vi "DMM_Scan PMPS 16V-15C Configure and Measure.vi"(0 "Scan Resources Handles In":T1, 5 "Scan Configuration":T5[](array[typedef]) {"Resolution in Digits" items=["3 1/2"=3.5, "4 1/2"=4.5, "5 1/2"=5.5, "6 1/2"=6.5, "7 1/2"=7.5]}, 11 "error in":errorcluster) -> (4 "Scan Resources Handles Out":T2, 6 "Formatted Measurements":T4[](array[typedef]) {"Switch Time" format="%#_3p"}, 8 "Raw Measurements":T3[](array[typedef]) {"Value" format="%#_8g"}, 10 "Execution Settings":T7[](array[typedef]) {"Function" items=["DC Volts"=1, "AC Volts"=2, "DC Current"=3, "AC Current"=4, "2-Wire Resistance"=5, "4-Wire Resistance"=101, "Frequency"=104, "Period"=105, "AC Volts DC Coupled"=1001, "Diode"=1002, "Waveform Voltage"=1003, "Waveform Current"=1004, "Capacitance"=1005, "Inductance"=1006, "Temperature"=108]; "Absolute\nResolution" format="%#_6p"; "Input Resistance\n(Ohm)" format="%#_6p"; "Range" format="%#_6p"; "Minimum\nFrequency (Hz)" format="%#_6p"; "Aperture\nTime (s)" format="%#_6p"; "Auto Range\nValue" format="%#_6p"; "Settle\nTime (s)" format="%#_6p"}, 14 "Total Scan Time (s)":dbl format="%#.3p", 15 "error out":errorcluster)   [LabVIEW 2021, in "DMM_Scan PXI Mux PXI Shunt 16V-15C.lvlib"]
doc: "Configures an NI-DMM Scan measurement list on the resource provided by the Scan Resource Handles In control according to each given Channel number (ex. ch0, ch1), Function/Range, Digits. \n\nReturns Formatted Measurements based on Channels, Measurements (string with units), Out of Range, Individual Measurement Time (including configuration, apperture and relay debounce).\n\nReturns Raw Measurements (numeric values) to be used and compared in a sequencer.\n\nReturns Execution Settings and Total Scan Time (s) for optimization, debugging and reporting"
uses:
  DMM_Scan PXI Mux PXI Shunt 16V-15C.lvlib
  Typedefs/Scan configuration.ctl
  <instrlib>/niDMM/nidmm.llb/niDMM Resolution in Digits.ctl
  Typedefs/Measurement values.ctl
  Typedefs/Formatted measurement.ctl
  DMM Mixed Measurements/DMM Mixed Meas Typedefs/DMM Execution Settings.ctl
  Typedefs/Scan Resource Handles Out.ctl
  Typedefs/Scan Resource Handles In.ctl
  DMM Mixed Measurements/DMM Mixed Meas Typedefs/Function Settings.ctl
  Static Digital Path Generation/Typedefs/Terminal and State Settings.ctl
  Common/Typedefs/Execution Options - Measure.ctl
  DMM Mixed Measurements/DMM_Mixed Measurement.lvlib
  Static Digital Path Generation/Switch_Static Digital Path Generation.lvlib
panel:
  # "Inputs"
  # "Outputs"
  # "Channels"
  # "Values"
  # "Units"
  # "Out of R."
  # "Channels"
  # "Measurements"
  # "Out of."
  # "Time"
  # "Channels"
  # "Functions/Range"
  # "Digits"
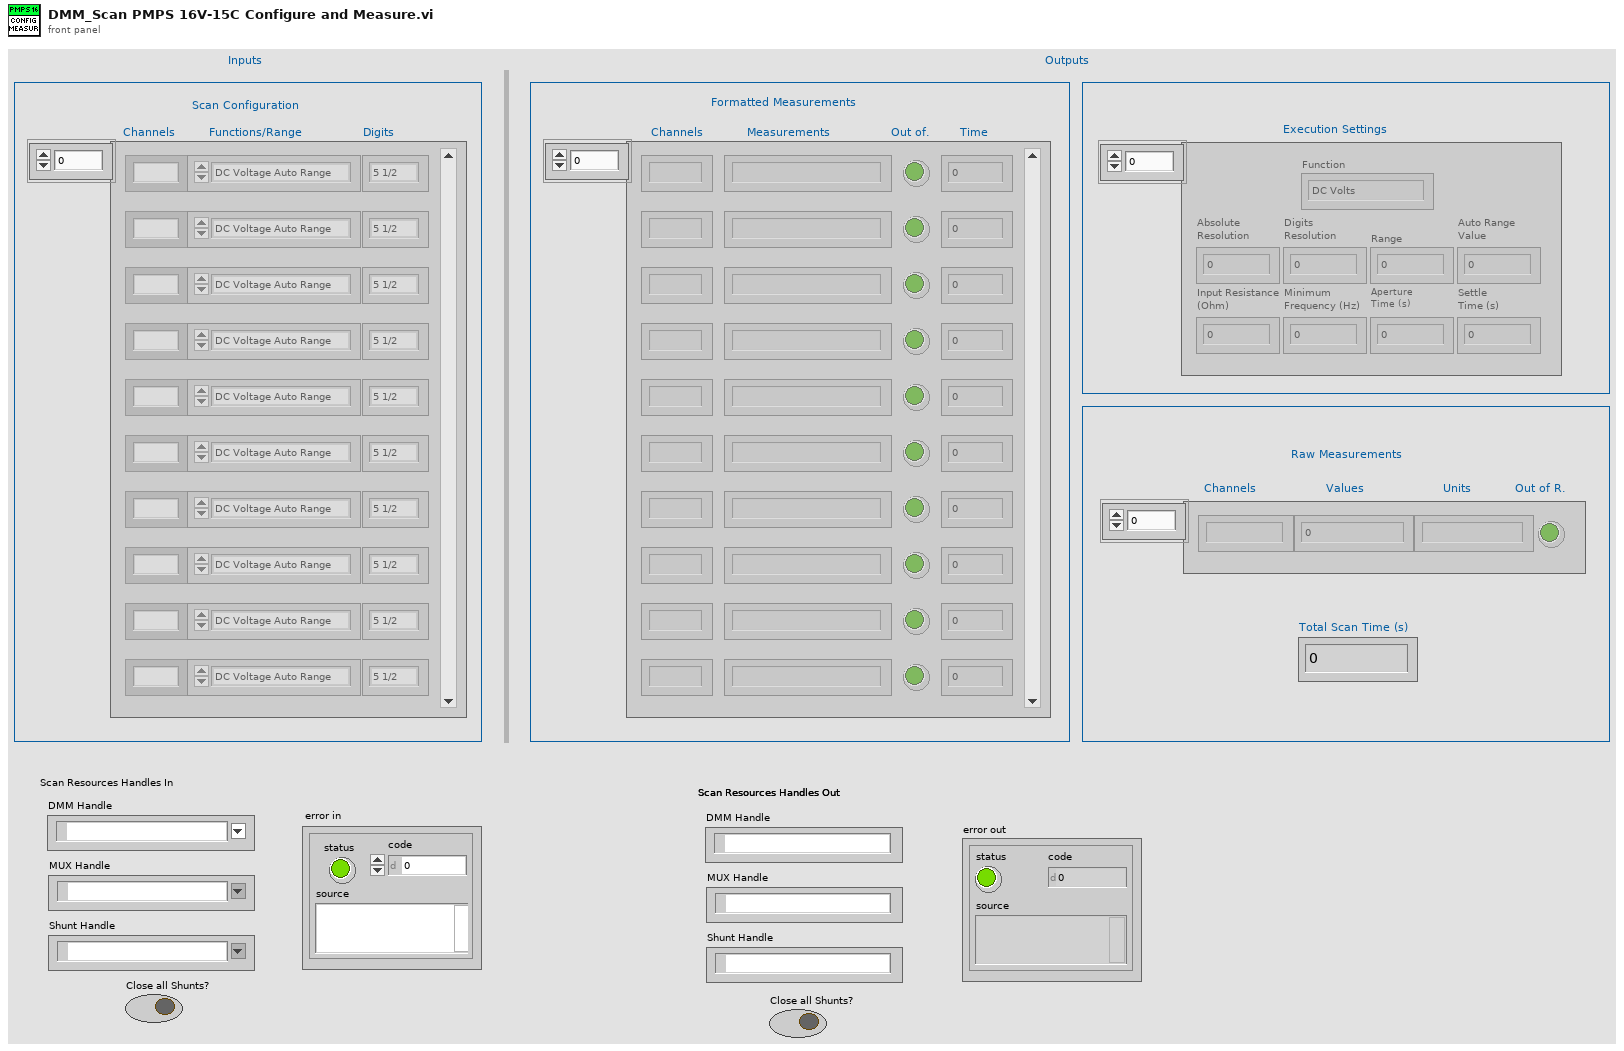
[diagram p1: front panel]
types:
  T1 = typedef "DMM_Scan PXI Mux PXI Shunt 16V-15C.lvlib/Scan Resource Handles In.ctl" = cluster{"DMM Handle":refnum<k15>, "MUX Handle":refnum<k15>, "Shunt Handle":refnum<k15>, "Close all Shunts?":bool}
  T2 = typedef "DMM_Scan PXI Mux PXI Shunt 16V-15C.lvlib/Scan Resource Handles Out.ctl" = cluster{"DMM Handle":refnum<k15>, "MUX Handle":refnum<k15>, "Shunt Handle":refnum<k15>, "Close all Shunts?":bool}
  T3 = typedef "DMM_Scan PXI Mux PXI Shunt 16V-15C.lvlib/Measurement values.ctl" = cluster{"Channel":string, "Value":dbl, "Unit":string, "Out of Range":bool}
  T4 = typedef "DMM_Scan PXI Mux PXI Shunt 16V-15C.lvlib/Formatted measurement.ctl" = cluster{"Channel":string, "Switch Time":dbl, "Formatted Measurement":string, "Out of Range":bool}
  T5 = typedef "DMM_Scan PXI Mux PXI Shunt 16V-15C.lvlib/Scan configuration.ctl" = cluster{"Channel":string, "Resolution in Digits":T6, "Range and Function":enum16{"DC Voltage Auto Range", "DC 100 mV", "DC 1 V ", "DC 10 V", "DC 100 V", "DC 300 V", " ", "AC Voltage Auto Range", "AC 50 mV", "AC 200 mV", "AC 500 mV", "AC 2 V", "AC 5 V", "AC 20 V", "AC 50 V", "AC 300 V", "  ", "DC Current Auto Range", "DC 1 uA", "DC 10 uA", "DC 100 uA", "DC 1 mA", "DC 10 mA", "DC 20 mA", "DC 100 mA", "DC 200 mA", "DC 1 A", "DC 3 A", "   ", "AC Current Auto Range", "AC 100 uA", "AC 1 mA", "AC 10 mA", "AC 100 mA", "AC 500 mA", "AC 1 A", "AC 3 A", "    ", "Resistance Auto Range", "Res 100 Ohm", "Res 1 kOhm", "Res 10 kOhm", "Res 100 kOhm", "Res 1 MOhm", "Res 10 MOhm", "Res 100 MOhm", "Res 5 GOhm", "     ", "Frequency AC Auto Range", "Freq AC 50 mV", "Freq AC 500 mV", "Freq AC 5 V", "Freq AC 50 V", "Freq AC 300 V", "      ", "Period AC Auto Range", "Period AC 50 mV", "Period AC 500 mV", "Period AC 5 V", "Period AC 50 V", "Period AC 300 V"}}
  T6 = typedef "niDMM Resolution in Digits.ctl" = dbl
  T7 = typedef "DMM_Mixed Measurement.lvlib/DMM Execution Settings.ctl" = cluster{"Absolute\nResolution":dbl, "Input Resistance\n(Ohm)":dbl, "Digits\nResolution":dbl, "Range":dbl, "Minimum\nFrequency (Hz)":dbl, "Aperture\nTime (s)":dbl, "Auto Range\nValue":dbl, "Settle\nTime (s)":dbl, "Function":i32}
  T8 = typedef "DMM_Mixed Measurement.lvlib/Function Settings.ctl" = cluster{"Range and Function":enum16{"DC Voltage Auto Range", "DC 100 mV", "DC 1 V ", "DC 10 V", "DC 100 V", "DC 300 V", " ", "AC Voltage Auto Range", "AC 50 mV", "AC 200 mV", "AC 500 mV", "AC 2 V", "AC 5 V", "AC 20 V", "AC 50 V", "AC 300 V", "  ", "DC Current Auto Range", "DC 1 uA", "DC 10 uA", "DC 100 uA", "DC 1 mA", "DC 10 mA", "DC 20 mA", "DC 100 mA", "DC 200 mA", "DC 1 A", "DC 3 A", "   ", "AC Current Auto Range", "AC 100 uA", "AC 1 mA", "AC 10 mA", "AC 100 mA", "AC 500 mA", "AC 1 A", "AC 3 A", "    ", "Resistance Auto Range", "Res 100 Ohm", "Res 1 kOhm", "Res 10 kOhm", "Res 100 kOhm", "Res 1 MOhm", "Res 10 MOhm", "Res 100 MOhm", "Res 5 GOhm", "     ", "Frequency AC Auto Range", "Freq AC 50 mV", "Freq AC 500 mV", "Freq AC 5 V", "Freq AC 50 V", "Freq AC 300 V", "      ", "Period AC Auto Range", "Period AC 50 mV", "Period AC 500 mV", "Period AC 5 V", "Period AC 50 V", "Period AC 300 V"}, "Resolution in Digits":T6}
  T9 = enum16{"DC Voltage Auto Range", "DC 100 mV", "DC 1 V ", "DC 10 V", "DC 100 V", "DC 300 V", " ", "AC Voltage Auto Range", "AC 50 mV", "AC 200 mV", "AC 500 mV", "AC 2 V", "AC 5 V", "AC 20 V", "AC 50 V", "AC 300 V", "  ", "DC Current Auto Range", "DC 1 uA", "DC 10 uA", "DC 100 uA", "DC 1 mA", "DC 10 mA", "DC 20 mA", "DC 100 mA", "DC 200 mA", "DC 1 A", "DC 3 A", "   ", "AC Current Auto Range", "AC 100 uA", "AC 1 mA", "AC 10 mA", "AC 100 mA", "AC 500 mA", "AC 1 A", "AC 3 A", "    ", "Resistance Auto Range", "Res 100 Ohm", "Res 1 kOhm", "Res 10 kOhm", "Res 100 kOhm", "Res 1 MOhm", "Res 10 MOhm", "Res 100 MOhm", "Res 5 GOhm", "     ", "Frequency AC Auto Range", "Freq AC 50 mV", "Freq AC 500 mV", "Freq AC 5 V", "Freq AC 50 V", "Freq AC 300 V", "      ", "Period AC Auto Range", "Period AC 50 mV", "Period AC 500 mV", "Period AC 5 V", "Period AC 50 V", "Period AC 300 V"}
  T10 = typedef "Execution Options - Measure.ctl" = enum16{"Configure & Measure", "Configure only", "Measure only"}
  T11 = typedef "Switch_Static Digital Path Generation.lvlib/Terminal and State Settings.ctl" = cluster{"Connect/Disconnect":bool, "Channel 1":string, "Channel 2":string}
  T12 = cluster{"Range and Function":bool, "Resolution in Digits":bool}
  T13 = typedef "DMM_Mixed Measurement.lvlib/Measurement.ctl" = cluster{"Measured Value":dbl, "Out of Range":bool, "Unit":string, "Measurement":string}
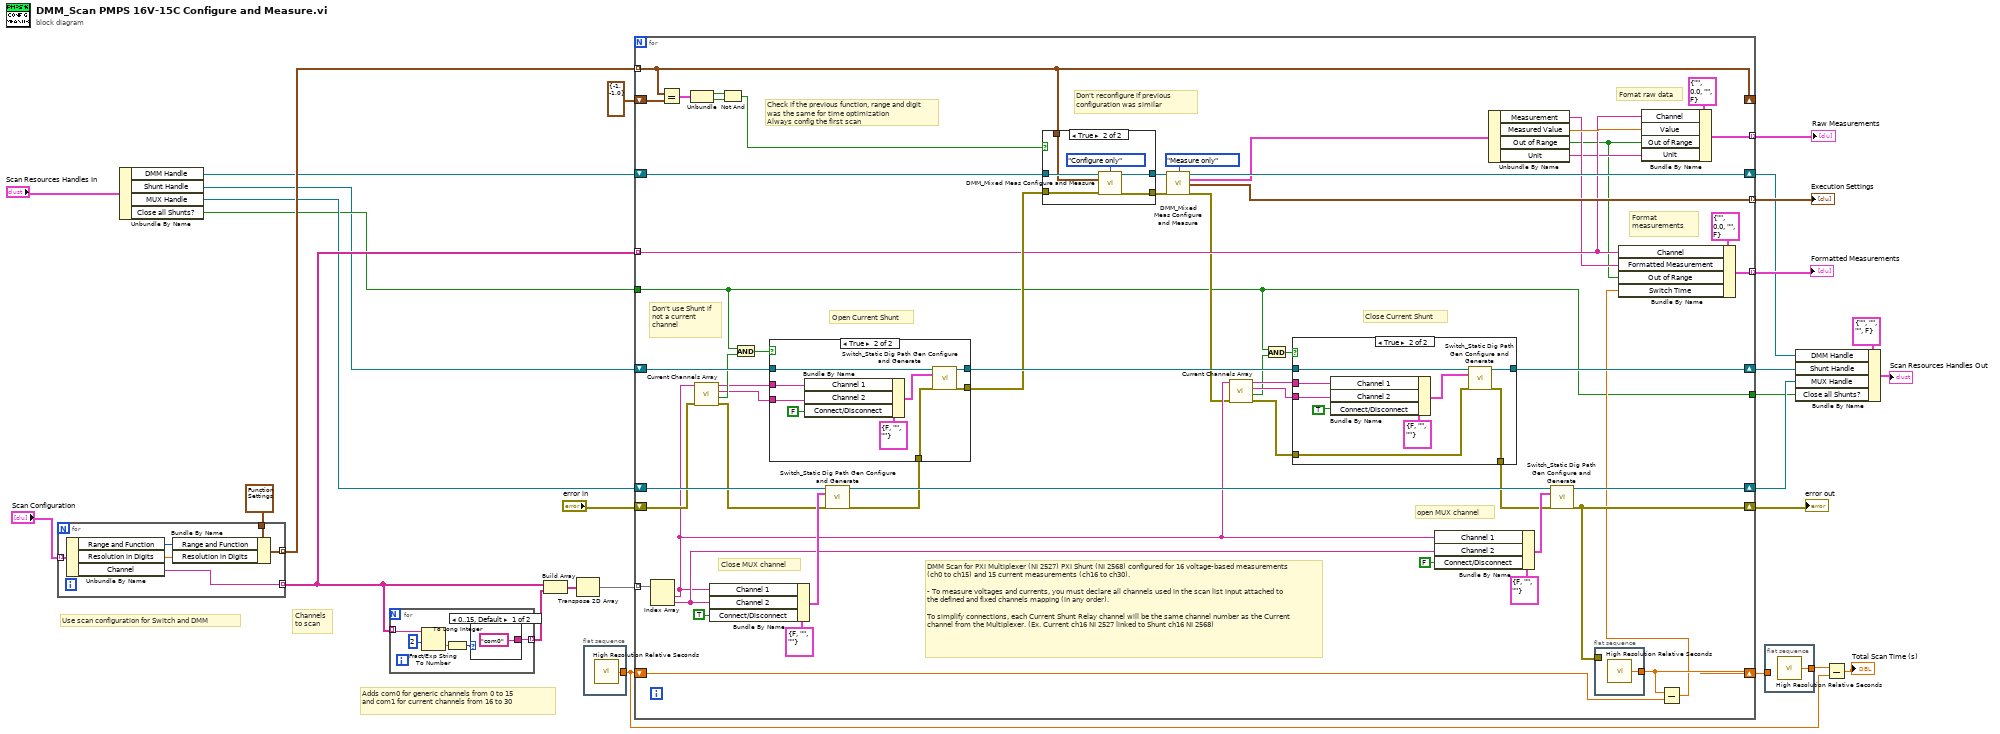
[diagram p0: block diagram]
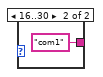
[diagram p2: hidden frame]
diagram:
  # "Adds com0 for generic channels from 0 to 15\nand com1 for current channels from 16 to 30"
  # "Use scan configuration for Switch and DMM"
  # "Channels\nto scan"
  n1 = for {
    tunnel: "Scan Configuration" -> [w33] mode=indexing
    tunnel: [w34] -> w20 mode=indexing
    tunnel: [w31] -> w28 mode=indexing
    tunnel: T8 {"Range and Function"=enum."DC Voltage Auto Range", "Resolution in Digits"=5.5} ("Function Settings") -> [w29]
    n2 = Unbundle By Name(w33) -> ("Range and Function"=w30:T9, "Resolution in Digits"=w32:T6, "Channel"=w34:string)
    n3 = Bundle By Name(cluster=w29, "Range and Function"=w30, "Resolution in Digits"=w32) -> (w31:T8)
  }
  n4 = Unbundle By Name("Scan Resources Handles In") -> ("DMM Handle"=w14:refnum<k15>, "Shunt Handle"=w8:refnum<k15>, "MUX Handle"=w13:refnum<k15>, "Close all Shunts?"=w10:bool)
  n5 = for {
    tunnel: [w37] -> w15 mode=indexing
    tunnel: w20 -> [w35] mode=indexing
    n6 = Fract/Exp String To Number(string=w35, offset=2 ("offset (0)")) -> (number=w38:dbl)  [unwired: 2 in, 1 out]
    n7 = To Long Integer(number=w38) -> (32bit integer=w36:i32)
    n8 = case shown="0..15, Default" w36 {
      tunnel: ["com0" "com1"] -> w37
      frame 0..15, Default {
      }
      frame 16..30 {
      }
    }
  }
  n9 = Build Array(w20, w15) -> (w16:string[][])
  n10 = Transpose 2D Array(2D array=w16) -> (transposed array=w22:string[][])
  n11 = flat-sequence {
    tunnel: [w42] -> w25
    frame #0 {
      n12 = call <vilib>:"High Resolution Relative Seconds.vi"() -> ("relative seconds"=w42:dbl)
    }
  }
  n13 = for {
    shift-right: [w97] -> w12
    shift-left: w14 -> [w84]
    shift-right: [w90] -> w2
    shift-left: w13 -> [w96]
    shift-right: [w91] -> w7
    shift-left: "error in" -> [w54]
    tunnel: w22 -> [w95] mode=indexing
    shift-right: [w99] -> w26
    shift-left: w25 -> [w98]
    shift-right: [w72] -> w3
    shift-left: w8 -> [w74]
    tunnel: w28 -> [w68] mode=indexing
    shift-right: [w68] -> _
    shift-left: cluster{i32, dbl} {-1, -1.0} -> [w75]
    tunnel: [w78] -> w17 mode=indexing
    tunnel: w20 -> [w62] mode=indexing
    tunnel: [w64] -> w19 mode=indexing
    tunnel: [w60] -> w18 mode=indexing
    tunnel: w10 -> [w43]
    tunnel: [w43] -> w1
    # "DMM Scan for PXI Multiplexer (NI 2527) PXI Shunt (NI 2568) configured for 16 voltage-based measurements (ch0 to ch15) and 15 current measurements (ch16 to ch30).\n\n- To measure voltages and currents, you must declare all channels used in the scan list input attached to the defined and fixed channels mapping (in any order). \n\nTo simplify connections, each Current Shunt Relay channel will be the same channel number as the Current channel from the Multiplexer. (Ex. Current ch16 NI 2527 linked to Shunt ch16 NI 2568)"
    # "Don't use Shunt if not a current channel"
    # "Format measurements"
    # "Fomat raw data"
    # "open MUX channel"
    # "Close MUX channel"
    # "Close Current Shunt"
    # "Open Current Shunt"
    # "Check if the previous function, range and digit was the same for time optimization\nAlways config the first scan"
    # "Don't reconfigure if previous configuration was similar"
    n14 = Index Array(array=w95) -> (element #1=w52:string, element #2=w88:string)  [unwired: 2 in]
    n15 = Equal?(x=w68, y=w75) -> (x = y?=w80:T12)
    n16 = Unbundle(w80) -> ("Range and Function"=w77:bool, "Resolution in Digits"=w76:bool)
    n17 = call "Current Channels Array.vi"("error in"=w54, "Channel 1"=w52) -> ("error out"=w53:errorcluster, "Current Channel?"=w49:bool, "Channel 2"=w47:string, "Channel 1"=w48:string)  [unwired: 6 in]
    n18 = Bundle By Name(cluster=T11 {"Connect/Disconnect"=FALSE, "Channel 1"="", "Channel 2"=""} ("Terminal and State Settings"), "Channel 1"=w52, "Channel 2"=w88, "Connect/Disconnect"=TRUE ("Connect Path")) -> (w94:T11)
    n19 = Not And(1:w76, 2:w77) -> (0:w79:bool)
    n20 = And(x=w43, y=w49) -> (x .and. y?=w56:bool)
    n21 = call "Switch_Static Dig Path Gen Configure and Generate.vi"("Switch Handle In"=w96, "Terminal and State Settings"=w94, "error in"=w53) -> ("Switch Handle Out"=w92:refnum<k15>, "error out"=w71:errorcluster)  [unwired: 10 in, 1 out]
    n22 = case shown="True" w56 {
      tunnel: w74 -> [w112 w121]
      tunnel: [w112 w120] -> w73
      tunnel: w71 -> [w111 w119]
      tunnel: [w111 w118] -> w70
      tunnel: w48 -> [_ w114]
      tunnel: w47 -> [_ w113]
      frame False {
      }
      frame True {
        n23 = Bundle By Name(cluster=T11 {"Connect/Disconnect"=FALSE, "Channel 1"="", "Channel 2"=""} ("Terminal and State Settings"), "Channel 1"=w114, "Channel 2"=w113, "Connect/Disconnect"=FALSE) -> (w117:T11)
        n24 = call "Switch_Static Dig Path Gen Configure and Generate.vi"("Switch Handle In"=w121, "Terminal and State Settings"=w117, "error in"=w119) -> ("Switch Handle Out"=w120:refnum<k15>, "error out"=w118:errorcluster)  [unwired: 10 in, 1 out]
      }
    }
    n25 = case shown="True" w79 {
      tunnel: w84 -> [w123 w129]
      tunnel: [w123 w128] -> w83
      tunnel: [w122 w126] -> w81
      tunnel: w68 -> [_ w124]
      tunnel: w70 -> [w122 w125]
      frame False {
      }
      frame True {
        n26 = call "DMM_Mixed Meas Configure and Measure.vi"("DMM Handle In"=w129, "Execution Option"=Execution_Options_-_Measure."Configure only", "Function Settings"=w124, "error in"=w125) -> ("DMM Handle Out"=w128:refnum<k15>, "error out"=w126:errorcluster)  [unwired: 8 in, 2 out]
      }
    }
    n27 = call "DMM_Mixed Meas Configure and Measure.vi"("DMM Handle In"=w83, "Execution Option"=Execution_Options_-_Measure."Measure only", "error in"=w81) -> ("DMM Handle Out"=w97:refnum<k15>, "Measurement"=w67:T13, "DMM Execution Settings"=w78:T7, "error out"=w51:errorcluster)  [unwired: 9 in]
    n28 = call "Current Channels Array.vi"("error in"=w51, "Channel 1"=w52) -> ("error out"=w50:errorcluster, "Current Channel?"=w44:bool, "Channel 2"=w45:string, "Channel 1"=w46:string)  [unwired: 6 in]
    n29 = And(x=w43, y=w44) -> (x .and. y?=w55:bool)
    n30 = case shown="True" w55 {
      tunnel: w73 -> [w101 w110]
      tunnel: [w101 w109] -> w72
      tunnel: [w100 w108] -> w69
      tunnel: w46 -> [_ w104]
      tunnel: w50 -> [w100 w103]
      tunnel: w45 -> [_ w102]
      frame False {
      }
      frame True {
        n31 = Bundle By Name(cluster=T11 {"Connect/Disconnect"=FALSE, "Channel 1"="", "Channel 2"=""} ("Terminal and State Settings"), "Channel 1"=w104, "Channel 2"=w102, "Connect/Disconnect"=TRUE) -> (w105:T11)
        n32 = call "Switch_Static Dig Path Gen Configure and Generate.vi"("Switch Handle In"=w110, "Terminal and State Settings"=w105, "error in"=w103) -> ("Switch Handle Out"=w109:refnum<k15>, "error out"=w108:errorcluster)  [unwired: 10 in, 1 out]
      }
    }
    n33 = Bundle By Name(cluster=T11 {"Connect/Disconnect"=FALSE, "Channel 1"="", "Channel 2"=""} ("Terminal and State Settings"), "Channel 1"=w52, "Channel 2"=w88, "Connect/Disconnect"=FALSE ("Disconnect Path")) -> (w89:T11)
    n34 = Unbundle By Name(w67) -> ("Measurement"=w61:string, "Measured Value"=w65:dbl, "Out of Range"=w58:bool, "Unit"=w59:string)
    n35 = call "Switch_Static Dig Path Gen Configure and Generate.vi"("Switch Handle In"=w92, "Terminal and State Settings"=w89, "error in"=w69) -> ("Switch Handle Out"=w90:refnum<k15>, "error out"=w91:errorcluster)  [unwired: 10 in, 1 out]
    n36 = flat-sequence {
      tunnel: [w130] -> w99
      tunnel: w91 -> [_]
      frame #0 {
        n37 = call <vilib>:"High Resolution Relative Seconds.vi"() -> ("relative seconds"=w130:dbl)
      }
    }
    n38 = Bundle By Name(cluster=T3 {"Channel"="", "Value"=0.0, "Unit"="", "Out of Range"=FALSE} ("Measurements"), "Channel"=w62, "Value"=w65, "Out of Range"=w58, "Unit"=w59) -> (w64:T3)
    n39 = Subtract(x=w99, y=w98) -> (x-y=w57:dbl)
    n40 = Bundle By Name(cluster=T4 {"Channel"="", "Switch Time"=0.0, "Formatted Measurement"="", "Out of Range"=FALSE} ("Measurements"), "Channel"=w62, "Formatted Measurement"=w61, "Out of Range"=w58, "Switch Time"=w57) -> (w60:T4)
  }
  "error out" <- w7
  "Raw Measurements" <- w19
  "Formatted Measurements" <- w18
  "Execution Settings" <- w17
  n41 = flat-sequence {
    tunnel: [w131] -> w24
    tunnel: w26 -> [_]
    frame #0 {
      n42 = call <vilib>:"High Resolution Relative Seconds.vi"() -> ("relative seconds"=w131:dbl)
    }
  }
  n43 = Bundle By Name(cluster=T2 {"DMM Handle"="", "MUX Handle"="", "Shunt Handle"="", "Close all Shunts?"=FALSE} ("Scan Resources Handles Out"), "DMM Handle"=w12, "Shunt Handle"=w3, "MUX Handle"=w2, "Close all Shunts?"=w1) -> (→"Scan Resources Handles Out":T2)
  n44 = Subtract(x=w24, y=w25) -> (x-y=→"Total Scan Time (s)":dbl)
